vi "Read Actual Position.vi"(4 "error in (no error)":errorcluster, 6 "Axis (1)":i32=1 min=1 max=3, 7 "VISA resource name":refnum<visa-resource-name>) -> (0 "error out":errorcluster, 1 "Returned string":string, 2 "Position (units)":dbl format="%.6g", 3 "VISA resource name out":refnum<visa-resource-name>)   [LabVIEW 2020, in "Newport ESP301.lvlib"]
doc: "Reads the current position.\nIt returns the instantaneous real position of the specified axis."
uses:
  Newport ESP301.lvlib
panel:
  out "concatenated string":string
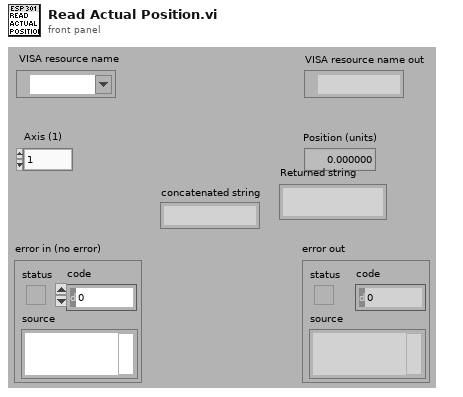
[diagram p1: front panel]
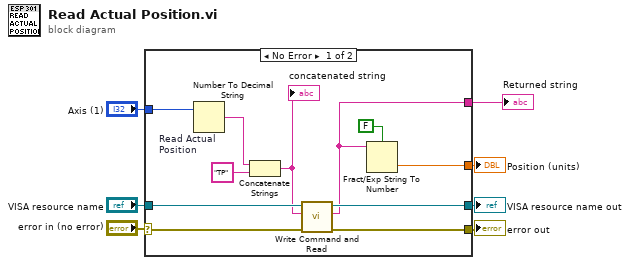
[diagram p0: block diagram]
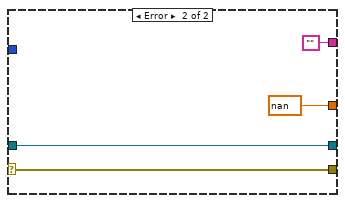
[diagram p2: hidden frame]
diagram:
  n1 = case shown="No Error" "error in (no error)" {
    selector: "error in (no error)" -> [w15 w22]
    tunnel: [w17 w22] -> w7
    tunnel: "VISA resource name" -> [w18 w21]
    tunnel: [w16 w21] -> w6
    tunnel: "Axis (1)" -> [w12 _]
    tunnel: [w10 nan] -> w2
    tunnel: [w8 ""] -> w1
    frame No Error {
      w14 = "TP"  # Read Actual Position
      n2 = Number To Decimal String(number=w12) -> (decimal integer string=w13:string)  [unwired: 1 in]
      n3 = Concatenate Strings(w13, w14) -> (w11:string)
      "concatenated string" <- w11
      n4 = call "Write Command and Read.vi"("error in (no error)"=w15, "Command"=w11, "VISA resource name"=w18) -> ("error out"=w17:errorcluster, "Returned string"=w8:string, "VISA resource name out"=w16:refnum<visa-resource-name>)  [unwired: 4 in]
      n5 = Fract/Exp String To Number(use system decimal point (T)=FALSE ("utiliser le séparateur décimal du système (V)"), string=w8) -> (number=w10:dbl)  [unwired: 2 in, 1 out]
    }
    frame Error {
    }
  }
  "error out" <- w7
  "VISA resource name out" <- w6
  "Position (units)" <- w2
  "Returned string" <- w1
